vi "Verify 0D DB Entries.vi"(11 "DB Entries":T1(array[cluster])) -> (2 "Cancelled?":bool, 3 "DB Entries Out":T1(array[cluster]))   [LabVIEW 2010]
panel:
  in  "System Cancel Button":bool
  in  "System OK Button":bool
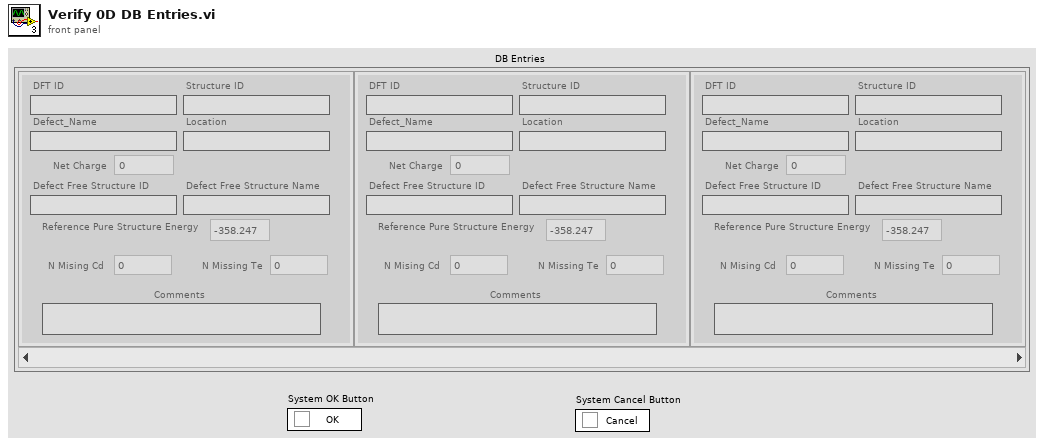
[diagram p1: front panel]
types:
  T1 = cluster{"DFT ID":string, "Structure ID":string, "Defect_Name":string, "Location":string, "Net Charge":i32, "Defect Free Structure ID":string, "Defect Free Structure Name":string, "Reference Pure Structure Energy":dbl, "N Mising Cd":i32, "N Missing Te":i32, "Comments":string}[]
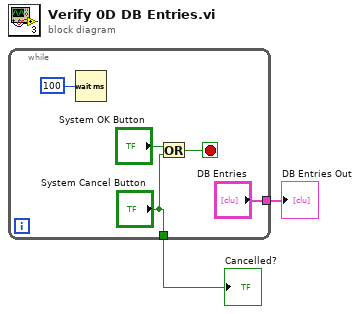
[diagram p0: block diagram]
diagram:
  n1 = while {
    tunnel: ["DB Entries"] -> w2
    tunnel: ["System Cancel Button"] -> w1
    stop <- w6 stop-if-true
    n2 = Wait (ms)(milliseconds to wait=u32 100) -> ()  [unwired: 1 out]
    n3 = Or(x="System OK Button", y="System Cancel Button") -> (x .or. y?=w6:bool)
  }
  "DB Entries Out" <- w2
  "Cancelled?" <- w1
